vi "SuperNS_Create.vi"(0 "reference in":refnum<class "SuperNS.lvclass">, 1 "NSName":string="CmdReader", 3 "RemoteEP_URL":string, 4 "Connection Lost Timeout (2000 ms)":i32=2000, 5 "error in (no error)":errorcluster, 6 "BufferSize (100)":i32=100, 7 "Element Allocation Mode":T1 caption="Element Allocation Mode (as needed)" items=["allocate as needed", "pre-allocate"], 8 "Writer (F: Reader)":bool, 9 "Low latency mode":T2(ring) caption="Low latency mode (None)", 10 "OpenProcessWindow(F)":bool, 11 "BG ConnCheck/Read period (200 ms)":i32=200) -> (14 "SuperNS Reference":refnum<class "SuperNS.lvclass">, 19 "error out":errorcluster)   [LabVIEW 2020, in "SuperNS.lvclass"]
doc: "Copyright © 2008 - 2024 VI Technologies B.V. \nALL RIGHTS RESERVED\n\n<b>Instantiates a SuperNS object.</b>\n\nDepending on the Writer input, internally creates the reader or writer endpoint of a network stream. The stream is of type LabVIEW Object (flattened to string).\n\nA SuperNS is an active object. It has a background process for stream (re)connecting and data reading.\n\nYou must always wire the <b>NSName</b> input. You should wire the <b>RemoteEP_URL</b> on only one of the endpoints to point to the other endpoint.\n\nCall the <b>GetReadDataEventRef</b> method to get an event registration refnum which you can use to retrieve the read data (for a reader endpoint) in an event structure.\n\nCall <b>WriteToStream</b> to write data to the stream (for a writer endpoint)\n\nSet <b>OpenProcess</b> input to true if you want to see the background process' frontpanel. You can always show/hide it at runtime by calling <b>OpenCloseThreadWin</b> method.\n\nAll other inputs are passed through to the network stream functions. See the LabVIEW help for more information on these.\n\nCall the <b>Destroy</b> method to destroy the object (and the network stream endpoint contained within).\n\nRefer to the Streaming Data and Sending Commands between Applications LabVIEW help topic for more information about using network streams."
uses:
  SuperNS.lvclass
  <vilib>/dex/Stream Element Allocation Mode.ctl
  StreamDataType.ctl
  <vilib>/dex/Flush And Wait Empty Condition.ctl
  SuperNS.lvclass/SuperNS.ctl
panel:
  # "Copyright (c) 2024, VI Technologies B.V.\nAll rights reserved.\n\nRedistribution and use in source and binary forms, with or without modification, are permitted provided that \nthe following conditions are met:\n\n * Redistributions of source code must retain the above copyright notice, this list of conditions and the \nfollowing disclaimer.\n * Redistributions in binary form must reproduce the above copyright notice, this list of conditions and the \nfollowing disclaimer in the documentation and/or other materials provided with the distribution.\n * Neither the name of VI Technologies B.V. nor the names of its contributors may be used to endorse or \npromote products derived from this software without specific prior written permission.\n\nTHIS SOFTWARE IS PROVIDED BY THE COPYRIGHT HOLDERS AND CONTRIBUTORS \"AS IS\" AND ANY EXPRESS OR \nIMPLIED WARRANTIES, INCLUDING, BUT NOT LIMITED TO, THE IMPLIED WARRANTIES OF MERCHANTABILITY \nAND FITNESS FOR A PARTICULAR PURPOSE ARE DISCLAIMED. IN NO EVENT SHALL THE COPYRIGHT OWNER OR \nCONTRIBUTORS BE LIABLE FOR ANY DIRECT, INDIRECT, INCIDENTAL, SPECIAL, EXEMPLARY, OR CONSEQUENTIAL \nDAMAGES (INCLUDING, BUT NOT LIMITED TO, PROCUREMENT OF SUBSTITUTE GOODS OR SERVICES; LOSS OF \nUSE, DATA, OR PROFITS; OR BUSINESS INTERRUPTION) HOWEVER CAUSED AND ON ANY THEORY OF LIABILITY, \nWHETHER IN CONTRACT, STRICT LIABILITY, OR TORT (INCLUDING NEGLIGENCE OR OTHERWISE) ARISING IN ANY \nWAY OUT OF THE USE OF THIS SOFTWARE, EVEN IF ADVISED OF THE POSSIBILITY OF SUCH DAMAGE.\n\nFor more information, please visit https://www.vi-tech.nl or contact us at info@vi-tech.nl"
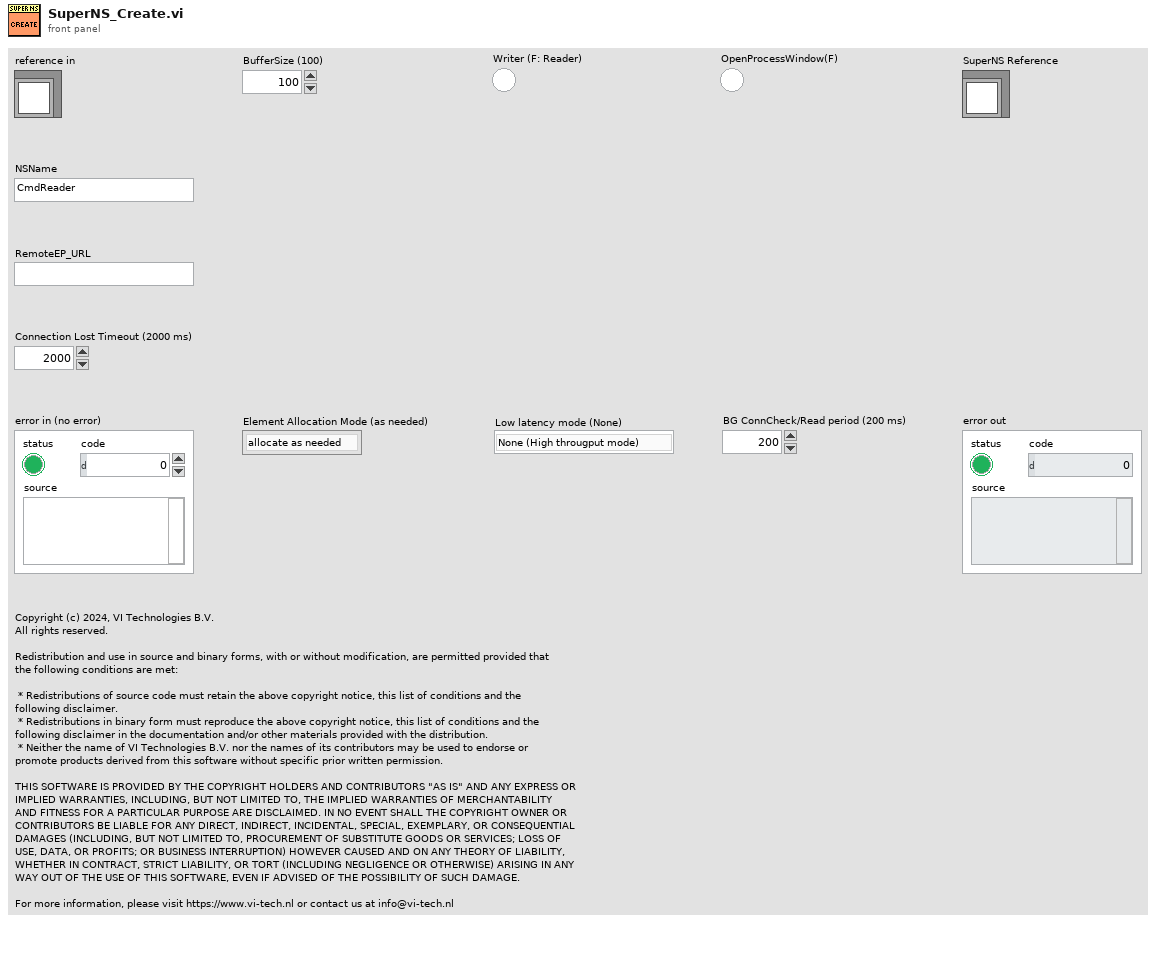
[diagram p1: front panel]
types:
  T1 = typedef "Stream Element Allocation Mode.ctl" = u32
  T2 = enum16{"None (High througput mode)", "All Elements Read From Stream", "All Elements Available for Reading"}
  T3 = typedef "SuperNS.lvclass/StreamDataType.ctl" = refnum<class>
  T4 = typedef "SuperNS.lvclass/ObjectAttributes.ctl" = cluster{"NSName":string, "RemoteEP_URL":string, "BufferSize":i32, "Element Allocation Mode":T1, "ConnLost Timeout":i32, "Writer":bool, "ReadDataEvent":string, "FlushAfterWrite":bool, "Thread":cluster{"VI Refnum":refnum<vi>, "Started Notifier":refnum<notifier>, "Stopped Notifier":refnum<notifier>, "CmdEvent":refnum<user-event>}, "Endpoint":refnum<k21>, "R/W Error":bool, "Flush Wait Condition":T5, "DataReadEvent":refnum<user-event>, "NS Created":bool, "BG ConnCheck/Read period":i32, "ErrorEvent":refnum<user-event>}
  T5 = typedef "Flush And Wait Empty Condition.ctl" = u8
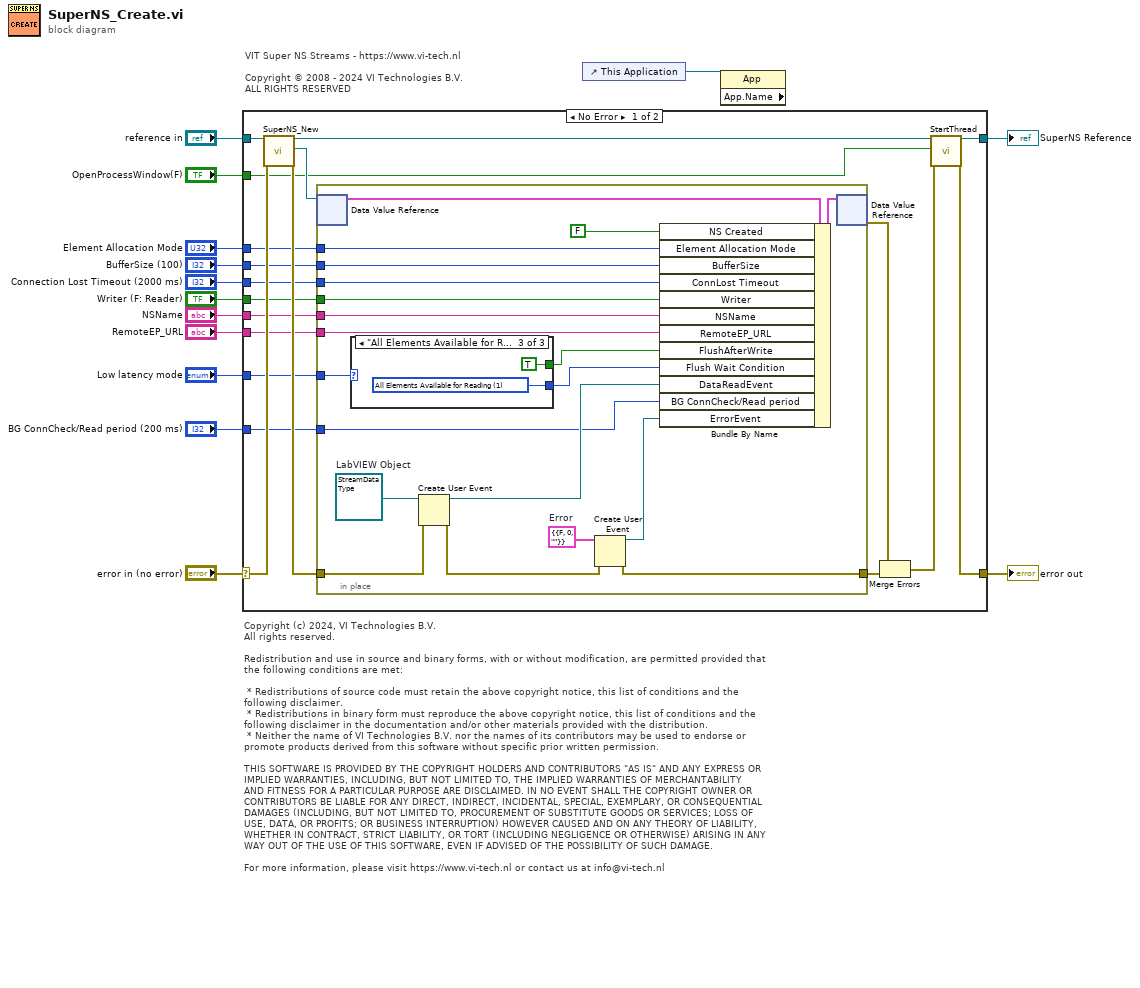
[diagram p0: block diagram]
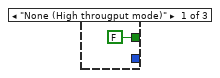
[diagram p2: hidden frame]
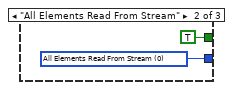
[diagram p3: hidden frame]
diagram:
  # "VIT Super NS Streams - https://www.vi-tech.nl\n\nCopyright © 2008 - 2024 VI Technologies B.V. \nALL RIGHTS RESERVED"
  # "Copyright (c) 2024, VI Technologies B.V.\nAll rights reserved.\n\nRedistribution and use in source and binary forms, with or without modification, are permitted provided that \nthe following conditions are met:\n\n * Redistributions of source code must retain the above copyright notice, this list of conditions and the \nfollowing disclaimer.\n * Redistributions in binary form must reproduce the above copyright notice, this list of conditions and the \nfollowing disclaimer in the documentation and/or other materials provided with the distribution.\n * Neither the name of VI Technologies B.V. nor the names of its contributors may be used to endorse or \npromote products derived from this software without specific prior written permission.\n\nTHIS SOFTWARE IS PROVIDED BY THE COPYRIGHT HOLDERS AND CONTRIBUTORS \"AS IS\" AND ANY EXPRESS OR \nIMPLIED WARRANTIES, INCLUDING, BUT NOT LIMITED TO, THE IMPLIED WARRANTIES OF MERCHANTABILITY \nAND FITNESS FOR A PARTICULAR PURPOSE ARE DISCLAIMED. IN NO EVENT SHALL THE COPYRIGHT OWNER OR \nCONTRIBUTORS BE LIABLE FOR ANY DIRECT, INDIRECT, INCIDENTAL, SPECIAL, EXEMPLARY, OR CONSEQUENTIAL \nDAMAGES (INCLUDING, BUT NOT LIMITED TO, PROCUREMENT OF SUBSTITUTE GOODS OR SERVICES; LOSS OF \nUSE, DATA, OR PROFITS; OR BUSINESS INTERRUPTION) HOWEVER CAUSED AND ON ANY THEORY OF LIABILITY, \nWHETHER IN CONTRACT, STRICT LIABILITY, OR TORT (INCLUDING NEGLIGENCE OR OTHERWISE) ARISING IN ANY \nWAY OUT OF THE USE OF THIS SOFTWARE, EVEN IF ADVISED OF THE POSSIBILITY OF SUCH DAMAGE.\n\nFor more information, please visit https://www.vi-tech.nl or contact us at info@vi-tech.nl"
  n1 = case shown="No Error" "error in (no error)" {
    selector: "error in (no error)" -> [w32 w60]
    tunnel: [w15 w60] -> w2
    tunnel: "reference in" -> [w33 w59]
    tunnel: [w27 w59] -> w13
    tunnel: "Writer (F: Reader)" -> [w26 _]
    tunnel: "NSName" -> [w25 _]
    tunnel: "RemoteEP_URL" -> [w24 _]
    tunnel: "Low latency mode" -> [w23 _]
    tunnel: "Element Allocation Mode" -> [w22 _]
    tunnel: "BufferSize (100)" -> [w21 _]
    tunnel: "Connection Lost Timeout (2000 ms)" -> [w20 _]
    tunnel: "OpenProcessWindow(F)" -> [w19 _]
    tunnel: "BG ConnCheck/Read period (200 ms)" -> [w18 _]
    frame No Error {
      n2 = call "SuperNS_New.vi"("reference in"=w33, "error in"=w32) -> ("reference out"=w28:refnum<class "SuperNS.lvclass">, "DVRRefOut"=w31:refnum<data-value>, "error out"=w30:errorcluster)  [unwired: 14 in, 1 out]
      n3 = in-place {
        in-place-border: w30 -> [w41]
        in-place-border: [w36] -> w29
        in-place-border: w26 -> [w51]
        in-place-border: w25 -> [w50]
        in-place-border: w24 -> [w49]
        in-place-border: w23 -> [w48]
        in-place-border: w22 -> [w45]
        in-place-border: w21 -> [w44]
        in-place-border: w20 -> [w43]
        in-place-border: w18 -> [w38]
        w35 = cluster{"error":errorcluster} {"error"={"status"=FALSE, "code"=0, "source"=""}}  # Error
        w42 = T3 refnum  # LabVIEW Object
        n4 = in-place-dvr #1(w31) -> (w52:T4)  [unwired: 1 out]
        n5 = case shown="\"All Elements Available for Reading\"" w48 {
          tunnel: [FALSE TRUE TRUE] -> w47
          tunnel: [_ w55 w57] -> w46
          frame "None (High througput mode)" {
          }
          frame "All Elements Read From Stream" {
            w55 = T5 0 items=["All Elements Read From Stream", "All Elements Available for Reading"] ("Flush Wait Condition")
          }
          frame "All Elements Available for Reading" {
            w57 = T5 1 items=["All Elements Read From Stream", "All Elements Available for Reading"] ("Flush Wait Condition")
          }
        }
        n6 = Create User Event(user event datatype=w42, error in=w41) -> (user event=w40:refnum<user-event>, error out=w37:errorcluster)
        n7 = Create User Event(user event datatype=w35, error in=w37) -> (user event=w34:refnum<user-event>, error out=w36:errorcluster)
        n8 = Bundle By Name(cluster=w52, "NS Created"=FALSE, "Element Allocation Mode"=w45, "BufferSize"=w44, "ConnLost Timeout"=w43, "Writer"=w51, "NSName"=w50, "RemoteEP_URL"=w49, "FlushAfterWrite"=w47, "Flush Wait Condition"=w46, "DataReadEvent"=w40, "BG ConnCheck/Read period"=w38, "ErrorEvent"=w34) -> (w53:T4)
        n9 = in-place-dvr #1(w53) -> (w17:errorcluster)  [unwired: 1 out]
      }
      n10 = Merge Errors(w17, w29) -> (w16:errorcluster)
      n11 = call "StartThread.vi"("reference in"=w28, "OpenThreadWin"=w19, "error in"=w16) -> ("reference out"=w27:refnum<class "SuperNS.lvclass">, "error out"=w15:errorcluster)  [unwired: 15 in]
    }
    frame Error {
    }
  }
  "SuperNS Reference" <- w13
  "error out" <- w2
  n12 = control-ref of="This Application"() -> (w3:refnum<vi>)
  n13 = property class="App" props=["App.Name"](reference=w3) -> ()  [unwired: 1 in, 3 out]
